vi "GEA2 Register for Multiple Events.vi"(0 "GEA2 Reference Array In":refnum<k24>[](array[refnum]), 11 "Error In":errorcluster) -> (4 "GEA2 Reference Array Out":refnum<k24>[](array[refnum]), 8 "GEA2 Event Registration":refnum<event-registration>, 15 "Error Out":errorcluster)   [LabVIEW 2014, in "GEA2_Toolkit.lvlib"]
doc: "This VI registers for events such that any messages that appear on the GEA2 bus trigger an event in LabVIEW. This event can be wired into an event structure and the message can be handled."
uses:
  library/GEA2_Toolkit.lvlib
  C:/Automation/DLLs/PC Tools .NET/GeaCommunication.dll
  Automation/DLLs/PC Tools .NET/GeaCommunication.dll
  type defs/Data Out.ctl
  GEA2 Message Event Handler.vi
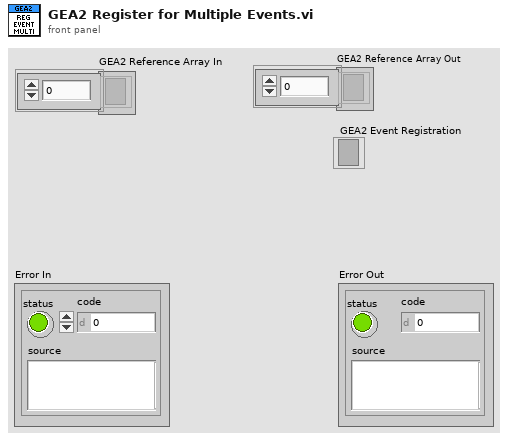
[diagram p1: front panel]
types:
  T1 = typedef "GEA2_Toolkit.lvlib/Data Out.ctl" = cluster{"Source":u8, "Destination":u8, "Command":u8, "Length":u8, "CRC":u16, "Message":string}
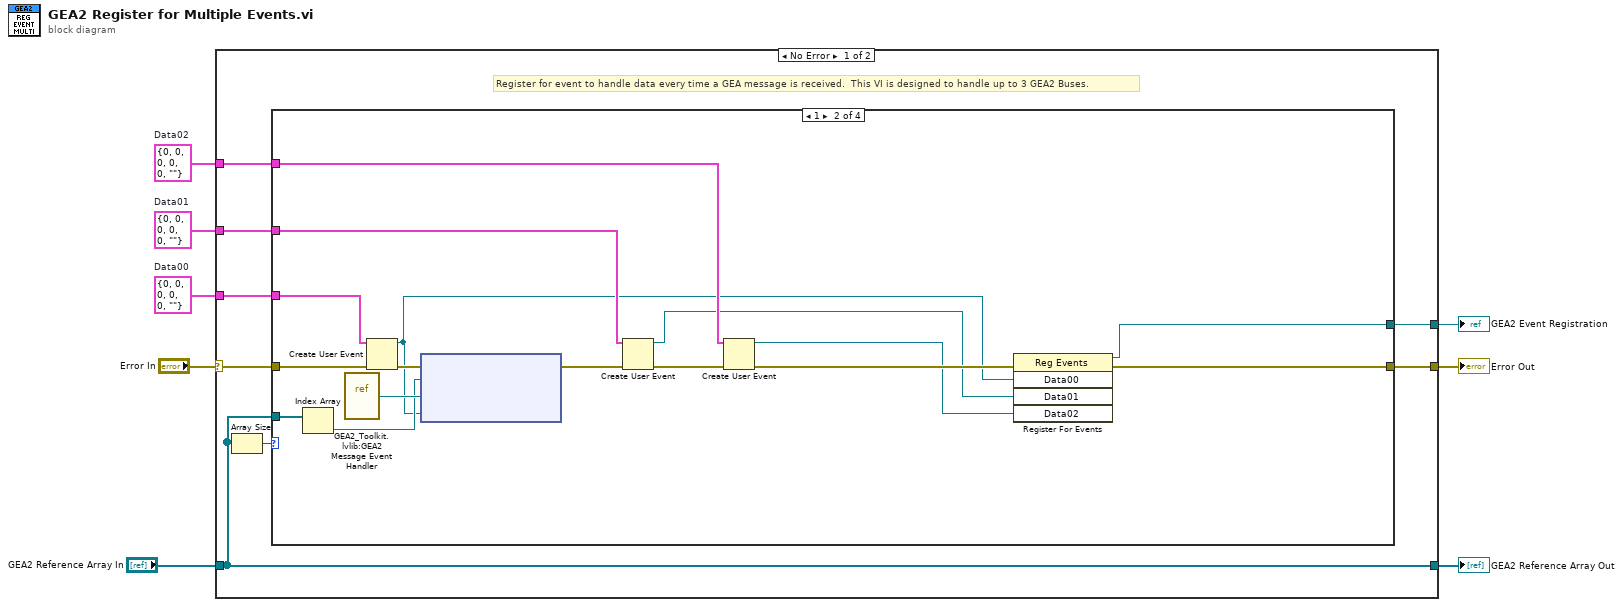
[diagram p0: block diagram]
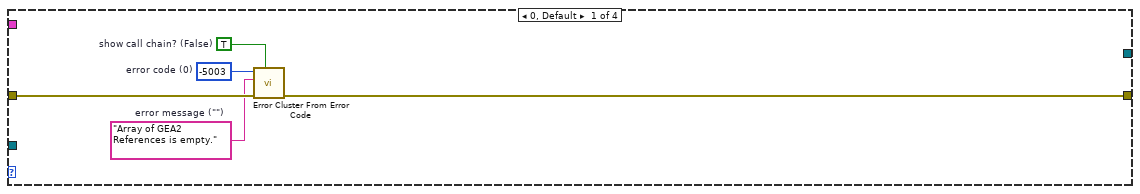
[diagram p2: hidden frame]
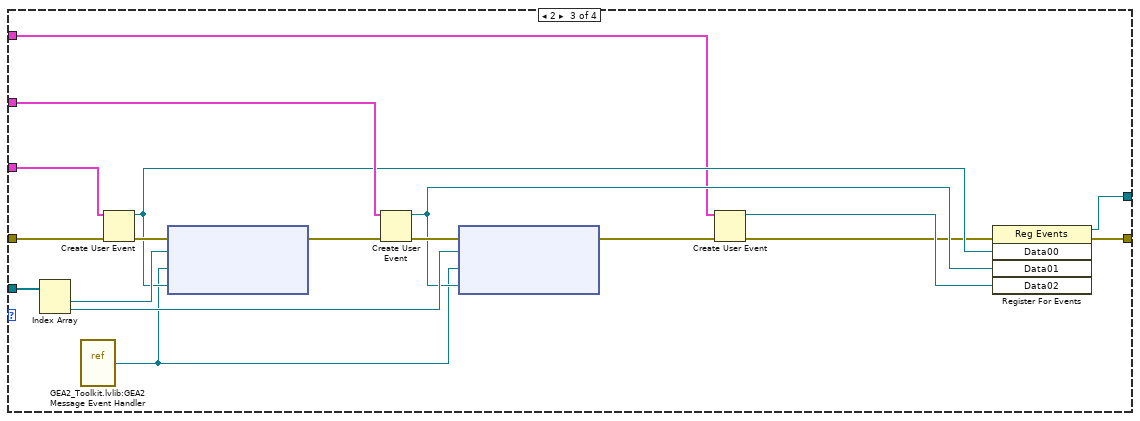
[diagram p3: hidden frame]
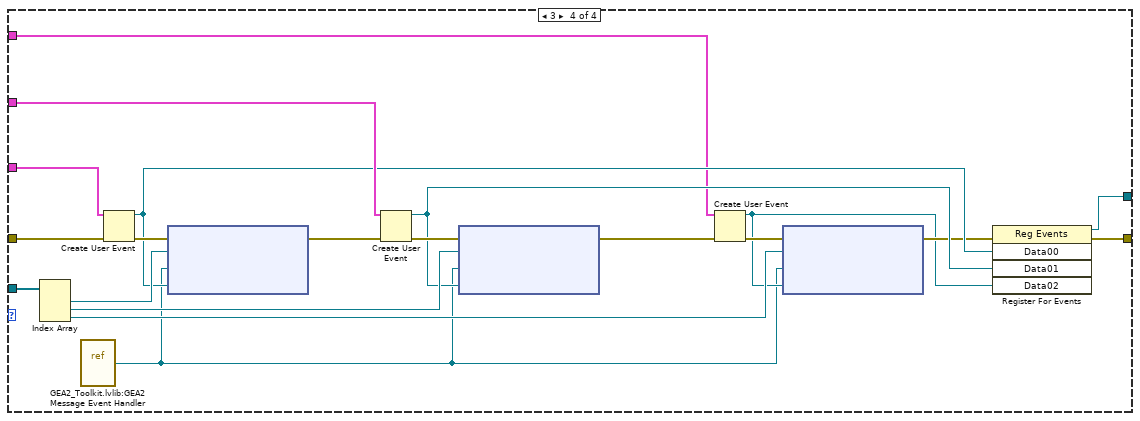
[diagram p4: hidden frame]
diagram:
  w2 = T1 {"Source"=0, "Destination"=0, "Command"=0, "Length"=0, "CRC"=0, "Message"=""}  # Data02
  w3 = T1 {"Source"=0, "Destination"=0, "Command"=0, "Length"=0, "CRC"=0, "Message"=""}  # Data01
  w7 = T1 {"Source"=0, "Destination"=0, "Command"=0, "Length"=0, "CRC"=0, "Message"=""}  # Data00
  n1 = case shown="No Error" "Error In" {
    selector: "Error In" -> [w15 w77]
    tunnel: [w16 w77] -> w8
    tunnel: w7 -> [w12 _]
    tunnel: "GEA2 Reference Array In" -> [w13 w76]
    tunnel: [w13 w76] -> w4
    tunnel: w3 -> [w11 _]
    tunnel: w2 -> [w10 _]
    tunnel: [w9 _] -> w1
    frame No Error {
      # "Register for event to handle data every time a GEA message is received.  This VI is designed to handle up to 3 GEA2 Buses."
      n2 = Array Size(array=w13) -> (size(s)=w14:i32)
      n3 = case shown="1" w14 {
        tunnel: [w17 w37 w55 w75] -> w16
        tunnel: w15 -> [w21 w36 w54 w74]
        tunnel: w13 -> [_ w33 w52 w72]
        tunnel: w12 -> [_ w26 w50 w70]
        tunnel: w11 -> [_ w27 w48 w68]
        tunnel: w10 -> [_ w28 w43 w63]
        tunnel: [_ w22 w39 w57] -> w9
        frame 0, Default {
          w18 = TRUE  # show call chain? (False)
          w19 = "Array of GEA2 References is empty."  # error message ("")
          w20 = -5003  # error code (0)
          n4 = call <vilib>:"Error Cluster From Error Code.vi"("show call chain? (False)"=w18, "error in (no error)"=w21, "error message (\"\")"=w19, "error code (0)"=w20) -> ("error out"=w17:errorcluster)  [unwired: 5 in]
        }
        frame 1 {
          n5 = Index Array(array=w33) -> (element=w32:refnum<k24>)  [unwired: 1 in]
          n6 = vi-ref "GEA2_Toolkit.lvlib:GEA2 Message Event Handler.vi"() -> (w34:refnum<vi>)
          n7 = Create User Event(user event datatype=w26, error in=w36) -> (user event=w25:refnum<user-event>, error out=w35:errorcluster)
          n8 = node(w35, w32, w34, w25) -> (w31:errorcluster)  [unwired: 1 in, 1 out]
          n9 = Create User Event(user event datatype=w27, error in=w31) -> (user event=w23:refnum<user-event>, error out=w30:errorcluster)
          n10 = Create User Event(user event datatype=w28, error in=w30) -> (user event=w24:refnum<user-event>, error out=w29:errorcluster)
          n11 = register-events(error in=w29, w25, w23, w24) -> (reference out=w22:refnum<event-registration>, error out=w37:errorcluster)  [unwired: 1 in]
        }
        frame 2 {
          n12 = Index Array(array=w52) -> (element #1=w51:refnum<k24>, element #2=w46:refnum<k24>)  [unwired: 2 in]
          n13 = vi-ref "GEA2_Toolkit.lvlib:GEA2 Message Event Handler.vi"() -> (w38:refnum<vi>)
          n14 = Create User Event(user event datatype=w50, error in=w54) -> (user event=w45:refnum<user-event>, error out=w53:errorcluster)
          n15 = node(w53, w51, w38, w45) -> (w49:errorcluster)  [unwired: 1 in, 1 out]
          n16 = Create User Event(user event datatype=w48, error in=w49) -> (user event=w44:refnum<user-event>, error out=w47:errorcluster)
          n17 = node(w47, w46, w38, w44) -> (w42:errorcluster)  [unwired: 1 in, 1 out]
          n18 = Create User Event(user event datatype=w43, error in=w42) -> (user event=w41:refnum<user-event>, error out=w40:errorcluster)
          n19 = register-events(error in=w40, w45, w44, w41) -> (reference out=w39:refnum<event-registration>, error out=w55:errorcluster)  [unwired: 1 in]
        }
        frame 3 {
          n20 = Index Array(array=w72) -> (element #1=w71:refnum<k24>, element #2=w66:refnum<k24>, element #3=w60:refnum<k24>)  [unwired: 3 in]
          n21 = vi-ref "GEA2_Toolkit.lvlib:GEA2 Message Event Handler.vi"() -> (w56:refnum<vi>)
          n22 = Create User Event(user event datatype=w70, error in=w74) -> (user event=w65:refnum<user-event>, error out=w73:errorcluster)
          n23 = node(w73, w71, w56, w65) -> (w69:errorcluster)  [unwired: 1 in, 1 out]
          n24 = Create User Event(user event datatype=w68, error in=w69) -> (user event=w64:refnum<user-event>, error out=w67:errorcluster)
          n25 = node(w67, w66, w56, w64) -> (w62:errorcluster)  [unwired: 1 in, 1 out]
          n26 = Create User Event(user event datatype=w63, error in=w62) -> (user event=w58:refnum<user-event>, error out=w61:errorcluster)
          n27 = node(w61, w60, w56, w58) -> (w59:errorcluster)  [unwired: 1 in, 1 out]
          n28 = register-events(error in=w59, w65, w64, w58) -> (reference out=w57:refnum<event-registration>, error out=w75:errorcluster)  [unwired: 1 in]
        }
      }
    }
    frame Error {
    }
  }
  "Error Out" <- w8
  "GEA2 Reference Array Out" <- w4
  "GEA2 Event Registration" <- w1
